vi "Drive Tasks.vi"(1 "Drive Task Parameters":T2) -> ()   [LabVIEW 2015]
uses:
  <vilib>/Rock Robotics/WPI/Utilities/WPI_GetSetVariantRefNum.vi
  Robot Global Data.vi
  <vilib>/Rock Robotics/WPI/RobotDrive/WPI_RobotDriveArcadeDrive_Standard(NoSaturation).vi
  <vilib>/Rock Robotics/Network Tables/NT Write Numeric Array.vi
panel:
  out "Centered Time":i32(graph)
  out "Gyro Rate":dbl
  out "Drive Operation":T1(ring)
  out "Set Point":dbl
  out "Current Gyro Value":dbl
  out "Iteration":i32
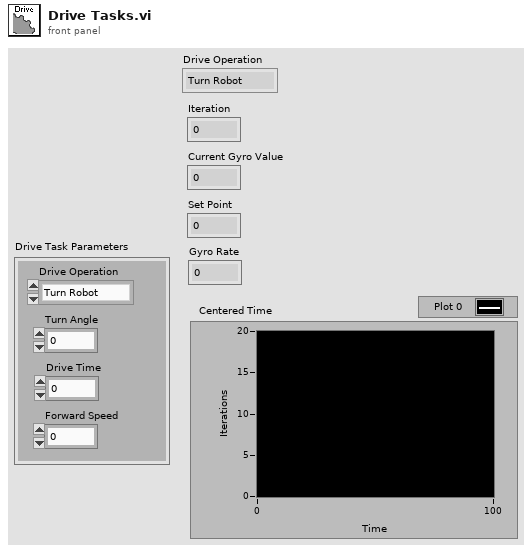
[diagram p1: front panel]
types:
  T1 = enum16{"Turn Robot", "Drive Straight for Time", "Drive to Obstacle Start"}
  T2 = cluster{"Turn Angle":dbl, "Drive Time":dbl, "Forward Speed":dbl, "Drive Operation":enum16{"Turn Robot", "Drive Straight for Time", "Drive to Obstacle Start"}}
  T3 = cluster{"X Angle":dbl, "Y Angle":dbl, "Z Angle":dbl}
  T4 = typedef "WPI_GyroDevRef.ctl" = cluster{"DevStatus":errorcluster, "Analog Channel":T5, "Offset":dbl, "Gain (VoltsPerDegree/Second)":dbl, "Gyro Type":enum16{"Analog", "XRS450"}, "Handle":i32, "SPI Bus":T6, "Device Found":bool, "Sample Rate":dbl, "Calibrate On Open":bool}
  T5 = typedef "FPGA_AIChannel.ctl" = enum8{"AI 0", "AI 1", "AI 2", "AI 3", "AI MXP 0", "AI MXP 1", "AI MXP 2", "AI MXP 3", "Invalid"}
  T6 = typedef "spi_bus.ctl" = enum16{"SPI On-Board, CS0", "SPI On-Board, CS1", "SPI On-Board, CS2", "SPI On-Board, CS3", "SPI MXP", "Invalid"}
  T7 = typedef "WPI_RobotDriveDevRef.ctl" = cluster{"DevStatus":errorcluster, "Motors[]":T8[], "Square Inputs":bool, "Max Output":dbl}
  T8 = typedef "WPI_MotorControlDeviceRef.ctl" = cluster{"DeviceStatus":errorcluster, "Type":T9, "PWM":cluster{"PWM Channel":T10, "DeadBand":T11}, "CAN":cluster{"Device Number":u8, "Control Mode":T12, "Semaphore":T13, "Max Vout":dbl, "TalonSRX Control Mode":T14}, "Invert":bool}
  T9 = typedef "WPI_MotorControlType.ctl" = enum16{"PWM", "CAN", "CANTalonSRX"}
  T10 = typedef "FPGA_DIOPWMChannel.ctl" = enum8{"PWM 0", "PWM 1", "PWM 2", "PWM 3", "PWM 4", "PWM 5", "PWM 6", "PWM 7", "PWM 8", "PWM 9", "PWM MXP 0", "PWM MXP 1", "PWM MXP 2", "PWM MXP 3", "PWM MXP 4", "PWM MXP 5", "PWM MXP 6", "PWM MXP 7", "PWM MXP 8", "PWM MXP 9", "Invalid"}
  T11 = typedef "WPI_PWMDeadband.ctl" = cluster{"Name":string, "maxPositivePwm":i32, "minPositivePwm":i32, "centerPwm":i32, "maxNegativePwm":i32, "minNegativePwm":i32, "angularRange":u16}
  T12 = typedef "WPI_CANJaguar_ControlMode.ctl" = enum8{"Percent VBus", "Current", "Speed", "Position", "Voltage"}
  T13 = typedef "Semaphore RefNum" = refnum<k1>
  T14 = typedef "WPI_CANTalonSRX_APIControlMode.ctl" = enum8{"Percent VBus", "Speed", "Position", "Slave", "Unchanged / Invalid", "Voltage Compensation", "Current", "Motion Profile"}
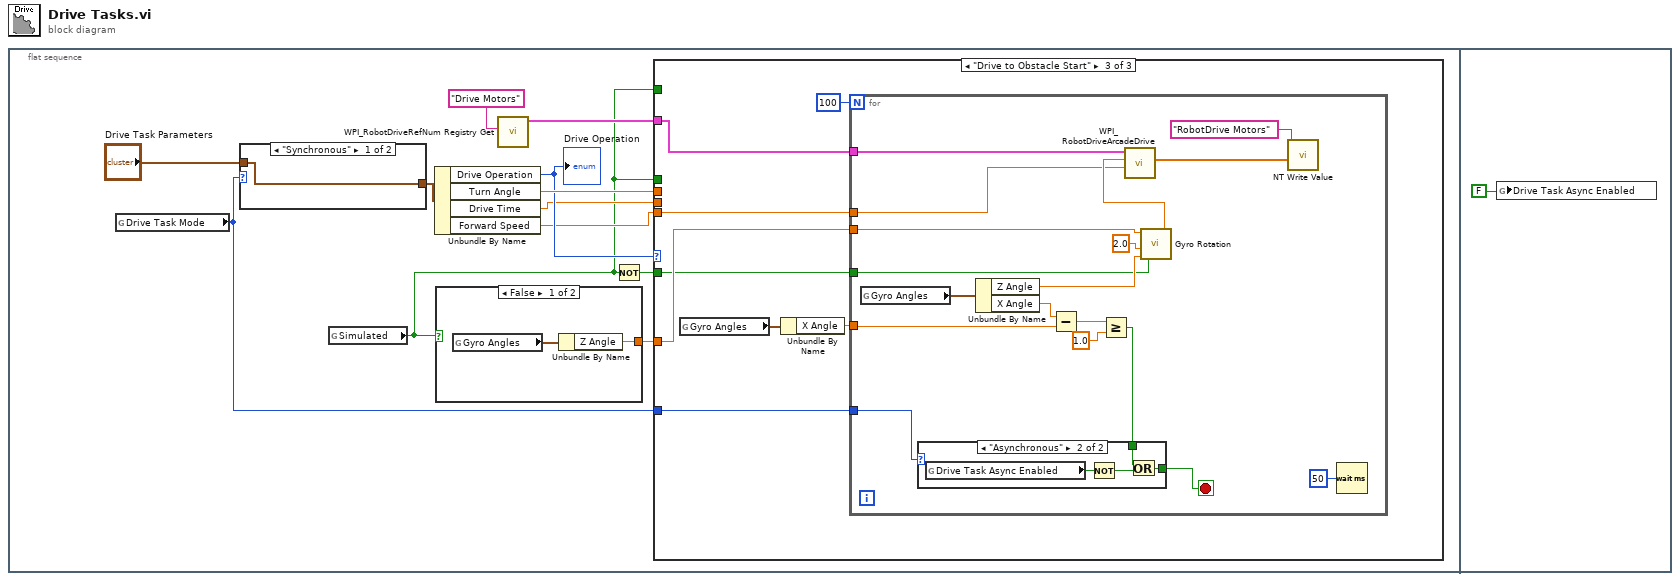
[diagram p0: block diagram]
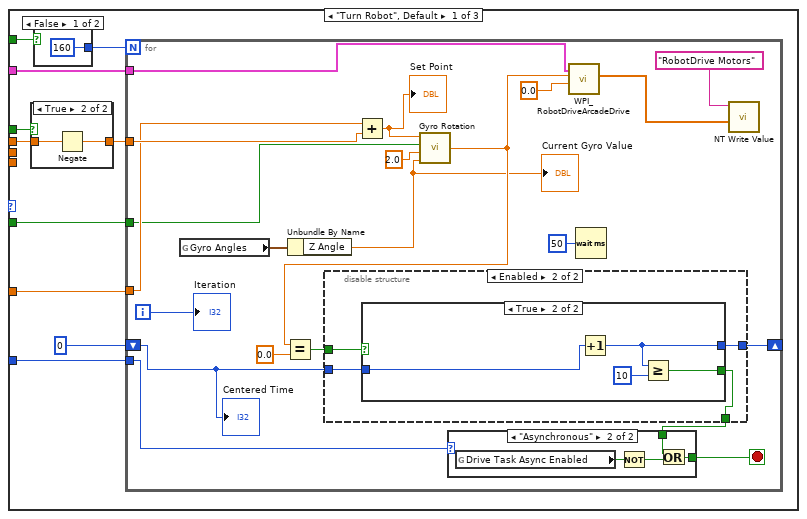
[diagram p2: hidden frame]
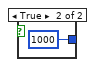
[diagram p4: hidden frame]
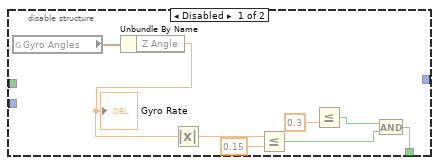
[diagram p5: hidden frame]
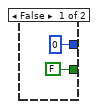
[diagram p6: hidden frame]
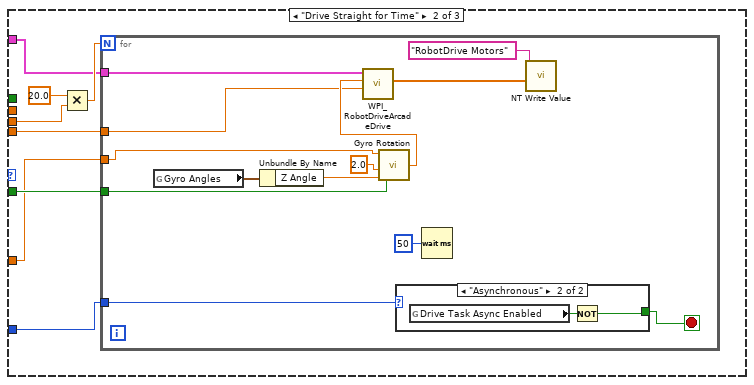
[diagram p8: hidden frame]
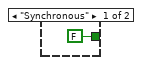
[diagram p9: hidden frame]
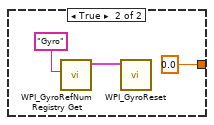
[diagram p11: hidden frame]
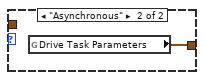
[diagram p12: hidden frame]
diagram:
  n1 = flat-sequence {
    frame #0 {
      n2 = global read "Robot Global Data.vi" "Drive Task Mode"() -> (w7:enum16{"Synchronous", "Asynchronous"})
      n3 = case shown="\"Synchronous\"" w7 {
        tunnel: [w133 w134] -> w10
        tunnel: "Drive Task Parameters" -> [w133 _]
        frame "Synchronous" {
        }
        frame "Asynchronous" {
          n4 = global read "Robot Global Data.vi" "Drive Task Parameters"() -> (w134:T2)
        }
      }
      n5 = global read "Robot Global Data.vi" "Simulated"() -> (w1:bool)
      n6 = Unbundle By Name(w10) -> ("Drive Operation"=w4:T1, "Turn Angle"=w9:dbl, "Drive Time"=w3:dbl, "Forward Speed"=w2:dbl)
      "Drive Operation" <- w4
      n7 = case shown="False" w1 {
        tunnel: [w128 0.0 ("Gyro Angle")] -> w6
        frame False {
          n8 = global read "Robot Global Data.vi" "Gyro Angles"() -> (w129:T3)
          n9 = Unbundle By Name(w129) -> ("Z Angle"=w128:dbl)
        }
        frame True {
          n10 = call <vilib>:"WPI_GyroRefNum Registry Get.vi"("refnum name"="Gyro") -> ("GyroDevRef"=w131:T4)  [unwired: 9 in, 1 out]
          n11 = call <vilib>:"WPI_GyroReset.vi"("GyroDevRef"=w131) -> ()  [unwired: 9 in, 2 out]
        }
      }
      n12 = call <vilib>:"WPI_RobotDriveRefNum Registry Get.vi"("refnum name"="Drive Motors") -> ("RobotDriveDevRef"=w11:T7)  [unwired: 1 in, 9 out]
      n13 = Not(x=w1) -> (.not. x?=w5:bool)
      n14 = case shown="\"Drive to Obstacle Start\"" w4 {
        tunnel: w11 -> [w21 w74 w102]
        tunnel: w9 -> [w14 _ _]
        tunnel: w7 -> [w20 w80 w98]
        tunnel: w6 -> [w19 w75 w101]
        tunnel: w5 -> [w18 w76 w97]
        tunnel: w3 -> [_ w79 _]
        tunnel: w2 -> [_ w73 w100]
        tunnel: w1 -> [w16 _ _]
        tunnel: w1 -> [w15 _ _]
        frame "Turn Robot", Default {
          n15 = case shown="True" w15 {
            tunnel: w14 -> [w23 w25]
            tunnel: [w23 w24] -> w13
            frame False {
            }
            frame True {
              n16 = Negate(x=w25) -> (-x=w24:dbl)
            }
          }
          n17 = case shown="False" w16 {
            tunnel: [160 1000] -> w22
            frame False {
            }
            frame True {
            }
          }
          n18 = for {
            N: w22 -> [_]
            tunnel: w21 -> [w47]
            tunnel: w13 -> [w42]
            tunnel: w19 -> [w40]
            tunnel: w20 -> [w36]
            tunnel: w18 -> [w35]
            shift-right: [w30] -> _
            shift-left: 0 -> [w29]
            i -> [w44]
            stop <- w39 stop-if-true
            n19 = global read "Robot Global Data.vi" "Gyro Angles"() -> (w41:T3)
            n20 = Unbundle By Name(w41) -> ("Z Angle"=w28:dbl)
            "Current Gyro Value" <- w28
            n21 = Add(x=w40, y=w42) -> (x+y=w45:dbl)
            "Set Point" <- w45
            n22 = call "Gyro Rotation.vi"("Current Value"=w28, "Deadband"=2.0, "Invert Rotation"=w35, "Set Point"=w45) -> ("Rotation"=w32:dbl)
            n23 = Equal?(x=w32, y=0.0) -> (x = y?=w31:bool)
            n24 = disable-structure shown="Enabled" {
              disable-tunnel: [w52 w58] -> w34
              disable-tunnel: w31 -> [_ w61]
              disable-tunnel: [_ w60] -> w30
              disable-tunnel: w29 -> [_ w59]
              frame Disabled {
                n25 = global read "Robot Global Data.vi" "Gyro Angles"() -> (w50:T3)
                n26 = Unbundle By Name(w50) -> ("Z Angle"=w49:dbl)
                "Gyro Rate" <- w49
                n27 = Absolute Value(x=w49) -> (abs(x)=w56:dbl)
                n28 = Less Or Equal?(x=w56, y=0.15) -> (x <= y?=w54:bool)
                n29 = Less Or Equal?(y=0.3) -> (x=w51:dbl, x <= y?=w53:bool)
                n30 = And(x=w53, y=w54) -> (x .and. y?=w52:bool)
              }
              frame Enabled {
                n31 = case shown="True" w61 {
                  tunnel: [0 w66] -> w60
                  tunnel: w59 -> [_ w67]
                  tunnel: [FALSE w64] -> w58
                  frame False {
                  }
                  frame True {
                    n32 = Increment(x=w67) -> (x+1=w66:i32)
                    n33 = Greater Or Equal?(x=w66, y=10) -> (x >= y?=w64:bool)
                  }
                }
              }
            }
            n34 = case shown="\"Asynchronous\"" w36 {
              tunnel: [w68 w72] -> w39
              tunnel: w34 -> [w68 w71]
              frame "Synchronous" {
              }
              frame "Asynchronous" {
                n35 = global read "Robot Global Data.vi" "Drive Task Async Enabled"() -> (w70:bool)
                n36 = Not(x=w70) -> (.not. x?=w69:bool)
                n37 = Or(x=w71, y=w69) -> (x .or. y?=w72:bool)
              }
            }
            n38 = call-poly <vilib>:"WPI_RobotDriveArcadeDrive.vi"("Y axis value"=0.0, "X axis value"=w32, "RobotDriveDevRef"=w47) -> ("Motor Values"=w37:dbl[])  [unwired: 6 in, 2 out]
            n39 = Wait (ms)(milliseconds to wait=u32 50) -> ()  [unwired: 1 out]
            n40 = call-poly <vilib>:"NT Write Value.vi"("Numeric Array"=w37, "Name"="RobotDrive Motors") -> ()  [unwired: 9 in, 1 out]
            "Iteration" <- w44
            "Centered Time" <- w29
          }
        }
        frame "Drive Straight for Time" {
          n41 = Multiply(x=20.0, y=w79) -> (x*y=w77:dbl)
          n42 = for {
            N: w77 -> [_]
            tunnel: w80 -> [w93]
            tunnel: w76 -> [w90]
            tunnel: w75 -> [w88]
            tunnel: w74 -> [w86]
            tunnel: w73 -> [w82]
            stop <- w92 stop-if-true
            n43 = global read "Robot Global Data.vi" "Gyro Angles"() -> (w87:T3)
            n44 = Unbundle By Name(w87) -> ("Z Angle"=w81:dbl)
            n45 = call "Gyro Rotation.vi"("Current Value"=w81, "Deadband"=2.0, "Invert Rotation"=w90, "Set Point"=w88) -> ("Rotation"=w85:dbl)
            n46 = call-poly <vilib>:"WPI_RobotDriveArcadeDrive.vi"("Y axis value"=w82, "X axis value"=w85, "RobotDriveDevRef"=w86) -> ("Motor Values"=w84:dbl[])  [unwired: 6 in, 2 out]
            n47 = case shown="\"Asynchronous\"" w93 {
              tunnel: [FALSE w95] -> w92
              frame "Synchronous" {
              }
              frame "Asynchronous" {
                n48 = global read "Robot Global Data.vi" "Drive Task Async Enabled"() -> (w96:bool)
                n49 = Not(x=w96) -> (.not. x?=w95:bool)
              }
            }
            n50 = Wait (ms)(milliseconds to wait=u32 50) -> ()  [unwired: 1 out]
            n51 = call-poly <vilib>:"NT Write Value.vi"("Numeric Array"=w84, "Name"="RobotDrive Motors") -> ()  [unwired: 9 in, 1 out]
          }
        }
        frame "Drive to Obstacle Start" {
          n52 = global read "Robot Global Data.vi" "Gyro Angles"() -> (w104:T3)
          n53 = Unbundle By Name(w104) -> ("X Angle"=w103:dbl)
          n54 = for {
            N: 100 -> [_]
            tunnel: w103 -> [w119]
            tunnel: w102 -> [w111]
            tunnel: w101 -> [w110]
            tunnel: w100 -> [w109]
            tunnel: w98 -> [w106]
            tunnel: w97 -> [w105]
            stop <- w122 stop-if-true
            n55 = global read "Robot Global Data.vi" "Gyro Angles"() -> (w121:T3)
            n56 = Unbundle By Name(w121) -> ("Z Angle"=w107:dbl, "X Angle"=w120:dbl)
            n57 = Subtract(x=w120, y=w119) -> (x-y=w118:dbl)
            n58 = Greater Or Equal?(x=w118, y=1.0) -> (x >= y?=w116:bool)
            n59 = case shown="\"Asynchronous\"" w106 {
              tunnel: [w123 w127] -> w122
              tunnel: w116 -> [w123 w126]
              frame "Synchronous" {
              }
              frame "Asynchronous" {
                n60 = global read "Robot Global Data.vi" "Drive Task Async Enabled"() -> (w125:bool)
                n61 = Not(x=w125) -> (.not. x?=w124:bool)
                n62 = Or(x=w126, y=w124) -> (x .or. y?=w127:bool)
              }
            }
            n63 = call "Gyro Rotation.vi"("Current Value"=w107, "Deadband"=2.0, "Invert Rotation"=w105, "Set Point"=w110) -> ("Rotation"=w114:dbl)
            n64 = call-poly <vilib>:"WPI_RobotDriveArcadeDrive.vi"("Y axis value"=w109, "X axis value"=w114, "RobotDriveDevRef"=w111) -> ("Motor Values"=w113:dbl[])  [unwired: 6 in, 2 out]
            n65 = call-poly <vilib>:"NT Write Value.vi"("Numeric Array"=w113, "Name"="RobotDrive Motors") -> ()  [unwired: 9 in, 1 out]
            n66 = Wait (ms)(milliseconds to wait=u32 50) -> ()  [unwired: 1 out]
          }
        }
      }
    }
    frame #1 {
      n67 = global write "Robot Global Data.vi" "Drive Task Async Enabled"(FALSE) -> ()
    }
  }
